vi "Log File Test.vi"() -> ()   [LabVIEW 2016]
doc: "--\nCopyright © 2017 Composed SystemsI All rights reserved.\n\nAuthor: Jon McBee <jon.mcbee@composed.io>\n\nThis library is provided \"AS IS\" ,WITHOUT WARRANTIES OR\nCONDITIONS OF ANY KIND, either express or implied.\n\nComposed Systems -- composed.io\n\nStream 0.0.1.1\nJon McBee - Composed Systems\nCopyright (c) 2017, Composed Systems"
uses:
  <vilib>/Composed Systems/Stream/Log/Text File Sink/Configuration.ctl
  <vilib>/Composed Systems/Stream/Log/Application Log/Log Level.ctl
  <vilib>/Composed Systems/Stream/Log/Asynchronous Application Log/Asynchronous Application Log.lvclass
  D:/Repos/Stream/.software/Log/Application Log/Application Log.lvclass
  <vilib>/Composed Systems/Stream/Log/CSV File Sink/CSV File Sink.lvclass/CSV File Sink.ctl
  <vilib>/Composed Systems/Stream/Log/String Control Sink/String Control Sink.lvclass
  D:/Repos/Stream/.software/Log/Log Sink/Log Sink.lvclass
  <vilib>/Composed Systems/Stream/Log/Text File Sink/Text File Sink.lvclass
  <vilib>/Composed Systems/Stream/Log/CSV File Sink/CSV File Sink.lvclass
  D:/Repos/Stream/.software/Log/Text File Sink/Text File Sink.lvclass
  <vilib>/Composed Systems/Stream/Log/Global Application Log/Global Application Log.lvclass
  <vilib>/Composed Systems/Stream/Log/Application Log/Application Log.lvclass
  <vilib>/Composed Systems/Stream/Error/Classes/Application Error/Application Error.lvclass
panel:
  in  "Message":string="Boom"
  in  "CSV File Sink Configuration":T1={"Folder"=path "D:/Temp/Log File Tester", "Name"="Comma", "Extension"="csv", "Mangle"=FALSE, "Append"=FALSE, "Flush"=FALSE, "Max Size (MB)"=100, "Timestamp Filename"=FALSE}
  out "String":string
  in  "error in (no error)":errorcluster
  in  "Bang":bool
  in  "Boom":bool
  in  "Text File Sink Configuration":T1={"Folder"=path "D:/Temp/Log File Tester", "Name"="Text", "Extension"="txt", "Mangle"=FALSE, "Append"=FALSE, "Flush"=FALSE, "Max Size (MB)"=100, "Timestamp Filename"=FALSE}
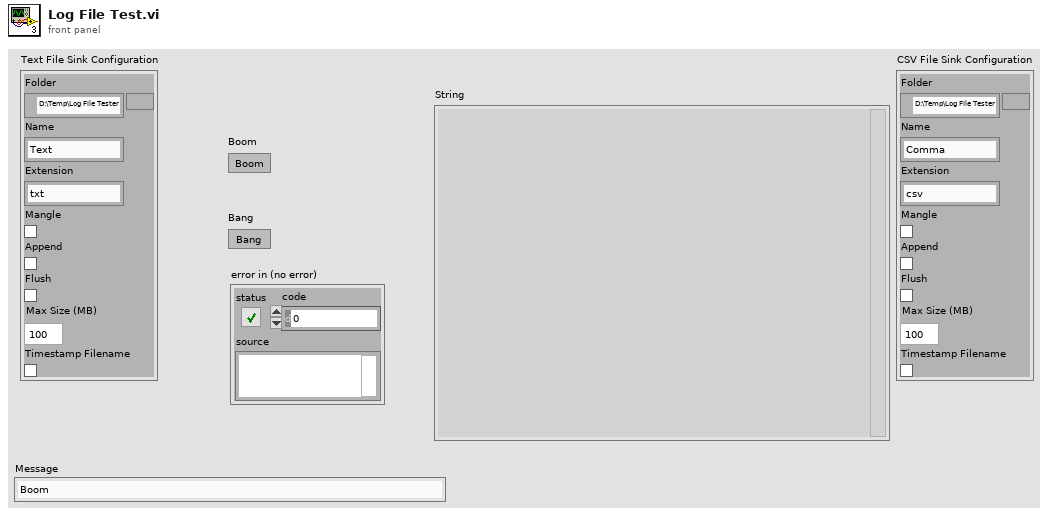
[diagram p1: front panel]
types:
  T1 = typedef "Stream Log.lvlib/Text File Sink.lvclass/Configuration.ctl" = cluster{"Folder":path, "Name":string, "Extension":string, "Mangle":bool, "Append":bool, "Flush":bool, "Max Size (MB)":i64, "Timestamp Filename":bool}
  T2 = typedef "Stream Log.lvlib/Application Log.lvclass/Log Level.ctl" = enum16{"Imperative", "Major", "Minor", "Debug", "Off"}
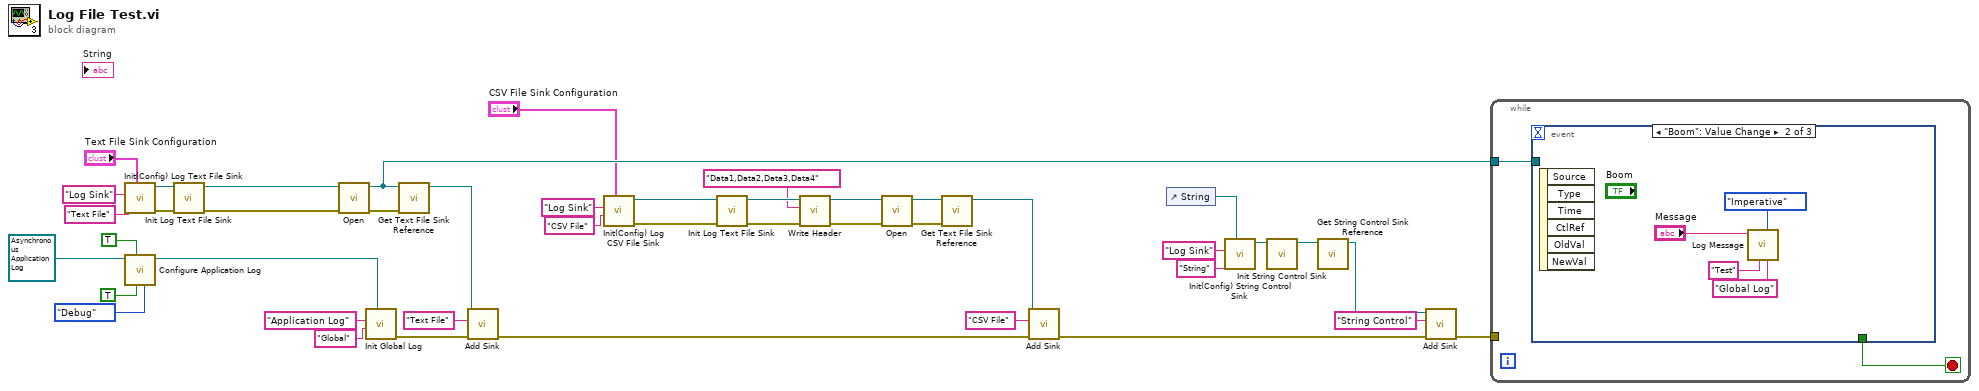
[diagram p0: block diagram]
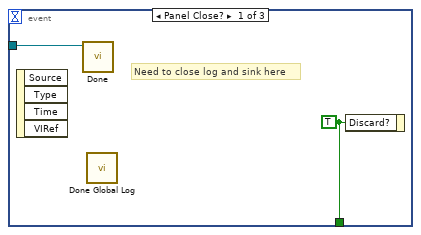
[diagram p2: hidden frame]
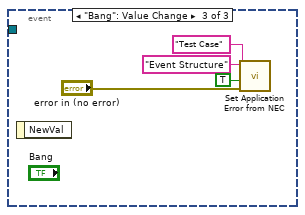
[diagram p3: hidden frame]
diagram:
  n1 = call <vilib>:"Init(Config) Log Text File Sink.vi"("Text File Sink Configuration"="Text File Sink Configuration", "iName"="Text File", "iType"="Log Sink") -> ("error out"=w40:errorcluster, "Text File Sink out"=w41:refnum<class "Text File Sink.lvclass">)  [unwired: 7 in]
  n2 = call-dynamic "Configure Application Log.vi"("Configuration.Level"=Log_Level."Debug", "Configuration.Enabled"=TRUE, "Configuration.Call Chain"=TRUE, "Asynchronous Application Log in"=refnum<class "Asynchronous Application Log.lvclass"> refnum ("Log.lvlib:Asynchronous Application Log.lvclass")) -> ("Asynchronous Application Log out"=w29:refnum<class "Asynchronous Application Log.lvclass">)  [unwired: 6 in, 1 out]
  n3 = call <vilib>:"Init Log Text File Sink.vi"("error in (no error)"=w40, "Text File Sink in"=w41) -> ("error out"=w39:errorcluster, "Text File Sink out"=w16:refnum<class "Text File Sink.lvclass">)  [unwired: 8 in]
  n4 = call <vilib>:"Open.vi"("error in (no error)"=w39, "Text File Sink in"=w16) -> ("error out"=w38:errorcluster, "Text File Sink out"=w30:refnum<class "Text File Sink.lvclass">)  [unwired: 8 in]
  n5 = call <vilib>:"Init Global Log.vi"("Application Log in"=w29, "iType"="Global", "iName"="Application Log") -> ("error out"=w42:errorcluster)  [unwired: 8 in]
  n6 = call <vilib>:"Get Text File Sink Reference.vi"("error in (no error)"=w38, "Text File Sink in"=w30) -> ("Text File Sink Reference"=w37:refnum<data-value>)  [unwired: 8 in, 1 out]
  n7 = call <vilib>:"Add Sink.vi"("error in (no error)"=w42, "Sink Name"="Text File", "Log Sink Reference"=w37) -> ("error out"=w14:errorcluster)  [unwired: 8 in]
  n8 = call <vilib>:"Init(Config) Log CSV File Sink.vi"("CSV File Sink Configuration"="CSV File Sink Configuration", "iName"="CSV File", "iType"="Log Sink") -> ("error out"=w8:errorcluster, "CSV File Sink"=w9:refnum<class "CSV File Sink.lvclass">)  [unwired: 7 in]
  n9 = call <vilib>:"Init Log Text File Sink.vi"("error in (no error)"=w8, "Text File Sink in"=w9) -> ("error out"=w10:errorcluster, "Text File Sink out"=w7:refnum<class "CSV File Sink.lvclass">)  [unwired: 8 in]
  n10 = call <vilib>:"Write Header.vi"("Header"="Data1,Data2,Data3,Data4", "CSV File Sink in"=w7) -> ("CSV File Sink out"=w6:refnum<class "CSV File Sink.lvclass">)  [unwired: 9 in]
  n11 = call <vilib>:"Open.vi"("error in (no error)"=w10, "Text File Sink in"=w6) -> ("error out"=w11:errorcluster, "Text File Sink out"=w12:refnum<class "CSV File Sink.lvclass">)  [unwired: 8 in]
  n12 = call <vilib>:"Get Text File Sink Reference.vi"("error in (no error)"=w11, "Text File Sink in"=w12) -> ("Text File Sink Reference"=w2:refnum<data-value>)  [unwired: 8 in, 1 out]
  n13 = call <vilib>:"Add Sink.vi"("error in (no error)"=w14, "Sink Name"="CSV File", "Log Sink Reference"=w2) -> ("error out"=w13:errorcluster)  [unwired: 8 in]
  n14 = control-ref of="String"() -> (w19:refnum<vi>)
  n15 = call <vilib>:"Init(Config) String Control Sink.vi"("Str Refnum"=w19, "iName"="String", "iType"="Log Sink") -> ("String Control Sink out"=w23:refnum<class "String Control Sink.lvclass">)  [unwired: 7 in, 1 out]
  n16 = call <vilib>:"Init String Control Sink.vi"("String Control Sink in"=w23) -> ("String Control Sink out"=w22:refnum<class "String Control Sink.lvclass">)  [unwired: 9 in, 1 out]
  n17 = call <vilib>:"Get String Control Sink Reference.vi"("String Control Sink in"=w22) -> ("data value reference"=w21:refnum<data-value>)  [unwired: 9 in, 1 out]
  n18 = call <vilib>:"Add Sink.vi"("error in (no error)"=w13, "Sink Name"="String Control", "Log Sink Reference"=w21) -> ("error out"=w24:errorcluster)  [unwired: 8 in]
  n19 = while {
    tunnel: w24 -> [_]
    tunnel: w30 -> [w43]
    stop <- w44 stop-if-true
    n20 = event shown="[1] \"Boom\": Value Change" {
      selector: _ -> [_ _ _]
      dyn-events: _ -> [_ _ _]
      timeout: _ -> [_ _ _]
      tunnel: [w46 _ _] -> w44
      tunnel: w43 -> [w45 _ _]
      event Panel Close? {
        w46 = TRUE ("Discard?")
        # "Need to close log and sink here"
        n21 = event-data() -> ()  [unwired: 1 in, 4 out]
        n22 = call-dynamic "Done.vi"("Text File Sink in"=w45) -> ()  [unwired: 9 in, 2 out]
        n23 = call <vilib>:"Done Global Log.vi"() -> ()  [unwired: 11 in, 1 out]
        n24 = event-data("Discard?"=w46) -> ()  [unwired: 1 in, 1 out]
      }
      event "Boom": Value Change {
        n25 = event-data() -> ()  [unwired: 1 in, 6 out]
        n26 = call <vilib>:"Log Message.vi"("Actor Name"="Global Log", "Level"=Log_Level."Imperative", "Actor Type"="Test", "Message"="Message") -> ()  [unwired: 7 in, 1 out]
      }
      event "Bang": Value Change {
        n27 = event-data() -> ()  [unwired: 1 in, 1 out]
        n28 = call <vilib>:"Set Application Error from NEC.vi"("Error In"="error in (no error)", "Log Error?"=TRUE, "Error Source"="Event Structure", "Error Scope"="Test Case") -> ()  [unwired: 7 in, 1 out]
      }
    }
  }
